vi "ClassifyExitPhoton.vi"(4 "WD (4)":dbl=4.0, 6 "NA (1)":dbl=1.0, 7 "n (1.33)":dbl=1.33, 9 "V - Exit":cluster{"X":dbl, "Y":dbl, "Z":dbl}={"X"=nan, "Y"=nan, "Z"=nan}, 10 "R - Exit":cluster{"X":dbl, "Y":dbl, "Z":dbl}={"X"=nan, "Y"=nan, "Z"=nan}, 11 "R - Focal Point":cluster{"X":dbl, "Y":dbl, "Z":dbl}={"X"=nan, "Y"=nan, "Z"=nan}) -> (2 "Phi":dbl, 3 "Photon State":T1)   [LabVIEW 2019]
uses:
  PhotonState--Enum.ctl
panel:
  out "Waveform Chart":dbl(graph)
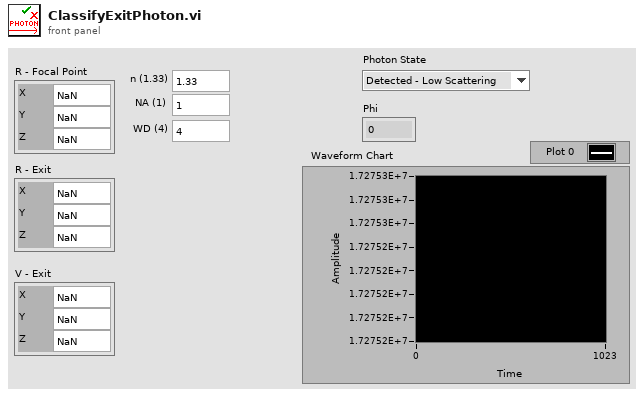
[diagram p1: front panel]
types:
  T1 = typedef "PhotonState--Enum.ctl" = enum16{"Detected - Low Scattering", "Detected - High Scattering", "Undetected"}
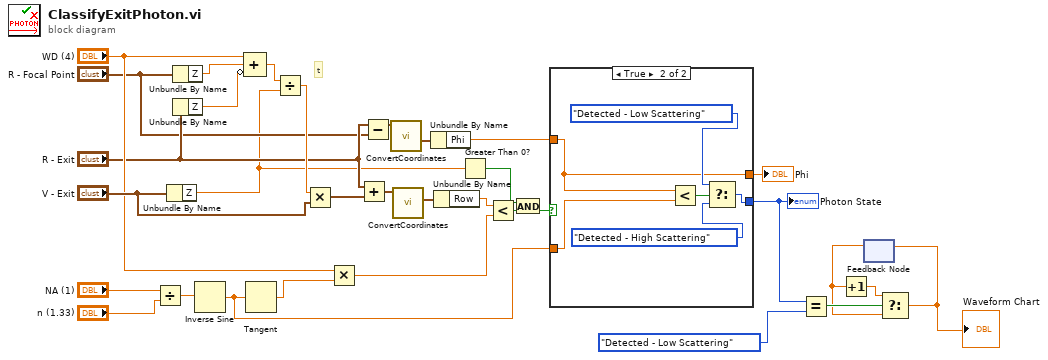
[diagram p0: block diagram]
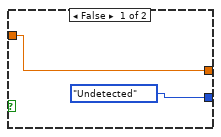
[diagram p2: hidden frame]
diagram:
  # "t"
  n1 = Divide(x="NA (1)", y="n (1.33)") -> (x/y=w22:dbl)
  n2 = Unbundle By Name("V - Exit") -> ("Z"=w7:dbl)
  n3 = Unbundle By Name("R - Focal Point") -> ("Z"=w32:dbl)
  n4 = Unbundle By Name("R - Exit") -> ("Z"=w31:dbl)
  n5 = Inverse Sine(1:w22) -> (0:w17:dbl)
  n6 = Compound Arithmetic op=ADD("WD (4)", w32, invert w31) -> (w30:dbl)
  n7 = Tangent(1:w17) -> (0:w21:dbl)
  n8 = Divide(x=w30, y=w7) -> (x/y=w28:dbl)
  n9 = Multiply(x=w28, y="V - Exit") -> (x*y=w10:cluster{"X":dbl, "Y":dbl, "Z":dbl})
  n10 = Multiply(x="WD (4)", y=w21) -> (x*y=w19:dbl)
  n11 = Add(x="R - Exit", y=w10) -> (x+y=w27:cluster{"X":dbl, "Y":dbl, "Z":dbl})
  n12 = Subtract(x="R - Exit", y="R - Focal Point") -> (x-y=w9:cluster{"X":dbl, "Y":dbl, "Z":dbl})
  n13 = call "ConvertCoordinates.vi"("XYZ Coordinates In"=w9) -> ("Spherical Coordinates Out"=w15:cluster{"R":dbl, "Theta":dbl, "Phi":dbl})  [unwired: 7 in, 3 out]
  n14 = call "ConvertCoordinates.vi"("XYZ Coordinates In"=w27) -> ("Cylindrical Coordinates Out"=w26:cluster{"Row":dbl, "Theta":dbl, "Z":dbl})  [unwired: 7 in, 3 out]
  n15 = Unbundle By Name(w15) -> ("Phi"=w13:dbl)
  n16 = Unbundle By Name(w26) -> ("Row"=w25:dbl)
  n17 = Greater Than 0?(x=w7) -> (x > 0?=w11:bool)
  n18 = Less?(x=w25, y=w19) -> (x < y?=w18:bool)
  n19 = And(x=w11, y=w18) -> (x .and. y?=w12:bool)
  n20 = case shown="True" w12 {
    tunnel: w17 -> [_ w40]
    tunnel: [PhotonState--Enum."Undetected" ("Photon State") w36] -> w6
    tunnel: [w33 w35] -> w16
    tunnel: w13 -> [w33 w35]
    frame False {
    }
    frame True {
      n21 = Less?(x=w35, y=w40) -> (x < y?=w39:bool)
      n22 = Select(t=PhotonState--Enum."Detected - Low Scattering" ("Photon State"), s=w39, f=PhotonState--Enum."Detected - High Scattering" ("Photon State")) -> (s? t:f=w36:T1)
    }
  }
  "Photon State" <- w6
  "Phi" <- w16
  n23 = Equal?(x=w6, y=PhotonState--Enum."Detected - Low Scattering" ("Photon State")) -> (x = y?=w4:bool)
  n24 = feedback #1() -> (w2:dbl)  [unwired: 1 in]
  n25 = Increment(x=w2) -> (x+1=w1:dbl)
  n26 = Select(t=w1, s=w4, f=w2) -> (s? t:f=w3:dbl)
  "Waveform Chart" <- w3
  n27 = feedback-in #1(w3) -> ()
